vi "Saturation.vi"(3 "Vmax":dbl=300.0 format="%#_13g", 4 "uk":dbl) -> (1 "real uk":dbl)   [LabVIEW 2015]
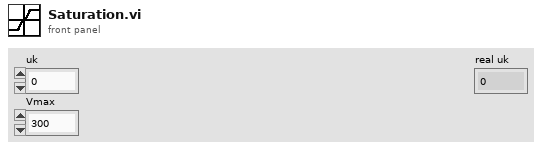
[diagram p1: front panel]
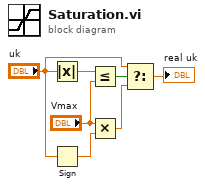
[diagram p0: block diagram]
diagram:
  n1 = Absolute Value(x="uk") -> (abs(x)=w7:dbl)
  n2 = Sign(1:"uk") -> (0:w3:dbl)
  n3 = Less Or Equal?(x=w7, y="Vmax") -> (x <= y?=w6:bool)
  n4 = Multiply(x="Vmax", y=w3) -> (x*y=w5:dbl)
  n5 = Select(t="uk", s=w6, f=w5) -> (s? t:f=→"real uk":dbl)
